vi "Configure Jitter Spectrum (More).vi"(0 "VISA resource name":refnum<visa-resource-name>, 1 "Enable Jitter Spectrum (Enable)":bool, 5 "Channel (1: Channel 1)":i32(ring) items=["Channel 1", "Channel 2", "Channel 3", "Channel 4", "Function 1", "Function 2", "Function 3", "Function 4", "Memory 1", "Memory 2", "Memory 3", "Memory 4"], 7 "Measurement Function (0: Rise Time)":i32(ring) items=["Rise Time", "Fall Time", "Frequency", "Period", "Width Negative", "Width Positive", "Duty Cycle Positive", "Cycle-cycle Duty Jitter(Rising)", "Cycle-cycle Duty Jitter(Falling)", "Cycle-cycle Jitter(Rising)", "Cycle-cycle Jitter(Falling)", "Cycle-cycle - Width", "Cycle-cycle + Width", "Data Rate", "Unit Interval", "Slew Rate", "Duty Cycle (Rising)", "Duty Cycle (Falling)"], 11 "error in (no error)":errorcluster) -> (4 "VISA resource name out":refnum<visa-resource-name>, 15 "error out":errorcluster)   [LabVIEW 2009, in "Agilent 8000 Series.lvlib"]
doc: "Configures a measurement and enables the Jitter Spectrum Jitter analysis on it.\n\n<B>Note:</B>\n(1)Calling this VI disables all previously enabled measurements and clears existing measurement results from display.\n\n(2)Duty cycle (rising) and Duty cycle (falling) have been added to the Measurement Function ring control. Data Rate and Unit Interval have their own VI (Configure Jitter Spectrum (Data Rate-Unit Interval)) which has added functionality."
uses:
  Agilent 8000 Series.lvlib
panel:
  # "Duty Cycle (rising) and \nDuty cycle (falling) are\n included in Measurement\nfunction ring."
  # "Data Rate and Unit \ninterval have a configure\nJitter Spectrum VI with\nadded functionality"
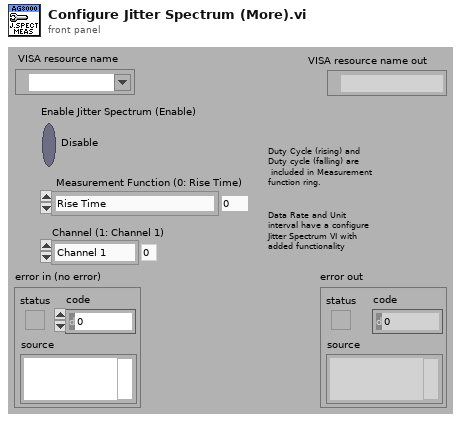
[diagram p1: front panel]
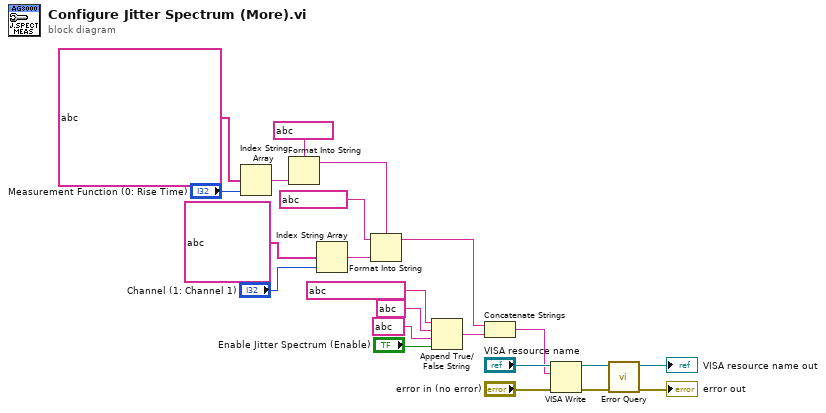
[diagram p0: block diagram]
diagram:
  n1 = Index String Array(1:"Measurement Function (0: Rise Time)", 2:string[] ?) -> (0:w13:string)  [unwired: 1 in]
  n2 = Format Into String(format string=string ?, w13) -> (resulting string=w12:string)  [unwired: 2 in, 1 out]
  n3 = Index String Array(1:"Channel (1: Channel 1)", 2:string[] ?) -> (0:w11:string)  [unwired: 1 in]
  n4 = Format Into String(format string=w12, initial string=string ?, w11) -> (resulting string=w4:string)  [unwired: 1 in, 1 out]
  n5 = Append True/False String(1:"Enable Jitter Spectrum (Enable)", 2:string ? ("false string"), 3:string ? ("true string"), 4:string ? ("string (\"\")")) -> (0:w5:string)
  n6 = Concatenate Strings(w4, w5) -> (w3:string)
  n7 = VISA Write(VISA resource name="VISA resource name", write buffer=w3, error in (no error)="error in (no error)") -> (VISA resource name out=w18:refnum<visa-resource-name>, error out=w17:errorcluster)  [unwired: 1 out]
  n8 = call "Error Query.vi"("error in (no error)"=w17, "VISA resource name"=w18) -> ("error out"=→"error out":errorcluster, "VISA resource name out"=→"VISA resource name out":refnum<visa-resource-name>)  [unwired: 6 in, 2 out]
